vi "Close.vi"(8 "error in (no error)":errorcluster, 11 "AsyncClassTemplate in":refnum<class "AsyncClassTemplate.lvclass">) -> (0 "error out":errorcluster)   [LabVIEW 2020, in "Vecto.lvlib" / "AsyncClassTemplate.lvclass"]
uses:
  AsyncClassTemplate.lvclass
  AsyncClassTemplate.lvclass/AsyncClassTemplate.ctl
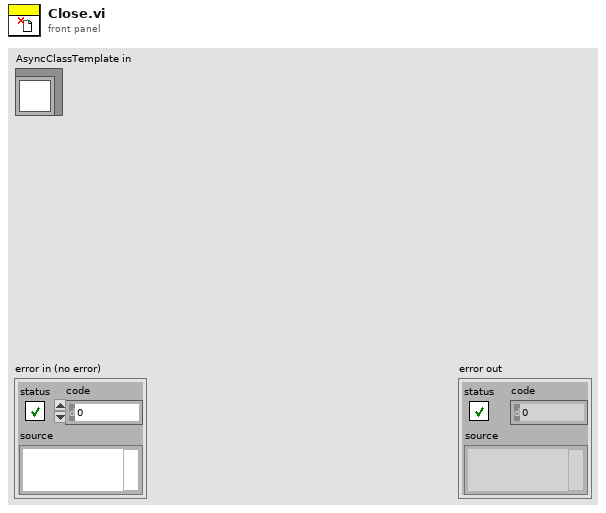
[diagram p1: front panel]
types:
  T1 = typedef "Vecto.lvlib/AsyncClassTemplate.lvclass/Incoming Events.ctl" = cluster{"Close":refnum<user-event>}
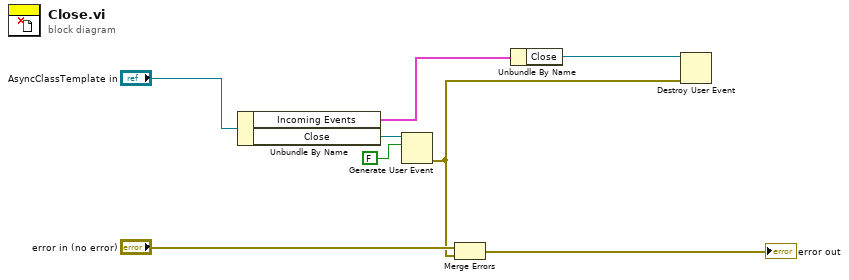
[diagram p0: block diagram]
diagram:
  n1 = Unbundle By Name("AsyncClassTemplate in") -> ("Incoming Events"=w4:T1, "Close"=w6:refnum<user-event>)
  n2 = Generate User Event(user event=w6, event data cluster=FALSE ("event data")) -> (error out=w1:errorcluster)  [unwired: 2 in, 1 out]
  n3 = Merge Errors("error in (no error)", w1) -> (→"error out":errorcluster)
  n4 = Unbundle By Name(w4) -> ("Close"=w3:refnum<user-event>)
  n5 = Destroy User Event(user event=w3, error in=w1) -> ()  [unwired: 1 out]
